vi "LS330_AddArray.vi"(9 "Array Cluster IN":T2, 10 "Queue IN":T4) -> (1 "Array Cluster OUT":T2, 2 "XY Plot Data":T1(array[cluster]))   [LabVIEW 2021]
uses:
  LS330_Status_Bundle.ctl
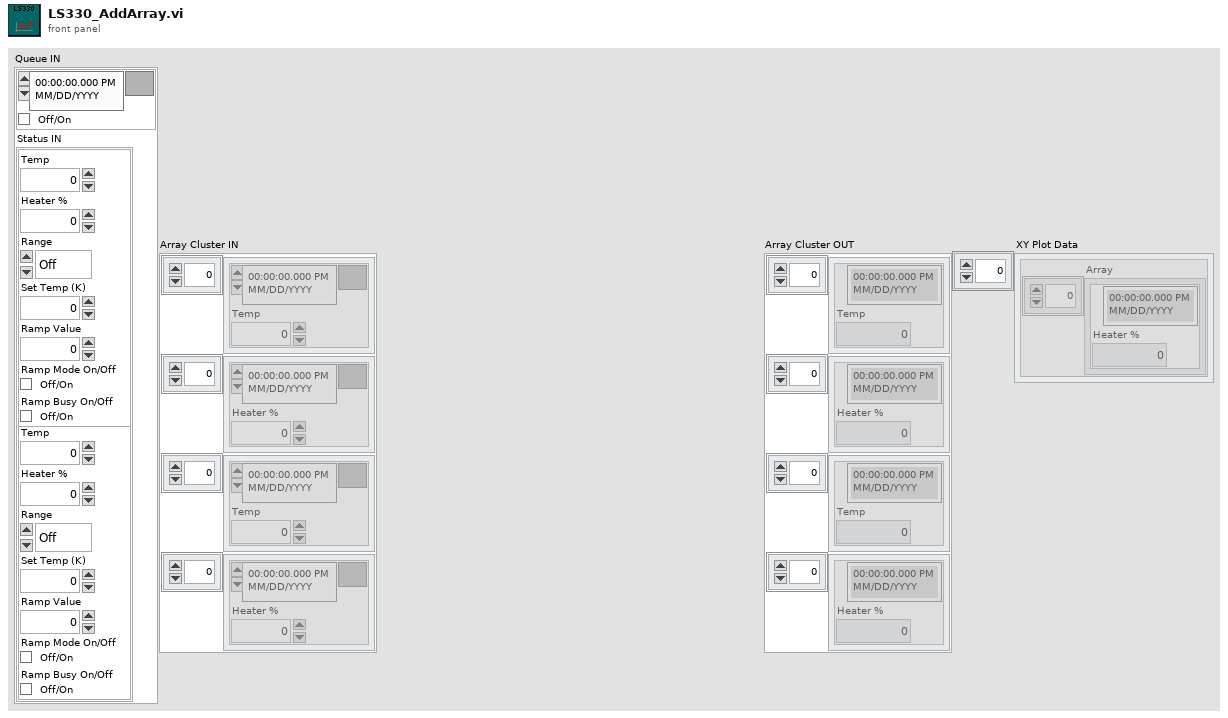
[diagram p1: front panel]
types:
  T1 = cluster{"Array":cluster{timestamp, "Heater %":dbl}[]}[]
  T2 = cluster{"Array":cluster{timestamp, "Temp":dbl}[], "Array":cluster{timestamp, "Heater %":dbl}[], "Array":cluster{timestamp, "Temp":dbl}[], "Array":cluster{timestamp, "Heater %":dbl}[]}
  T3 = typedef "LS330_Status_Bundle.ctl" = cluster{"Temp":dbl, "Heater %":dbl, "Range":enum16{"Off", "Low", "Medium", "High"}, "Set Temp (K)":dbl, "Ramp Value":dbl, "Ramp Mode On/Off":bool, "Ramp Busy On/Off":bool}
  T4 = cluster{"Cluster":cluster{timestamp, "Checkbox":bool}, "Status IN":cluster{T3, T3}}
  T5 = cluster{"Array":cluster{timestamp, "Temp":dbl}[]}
  T6 = cluster{"Array":cluster{timestamp, "Heater %":dbl}[]}
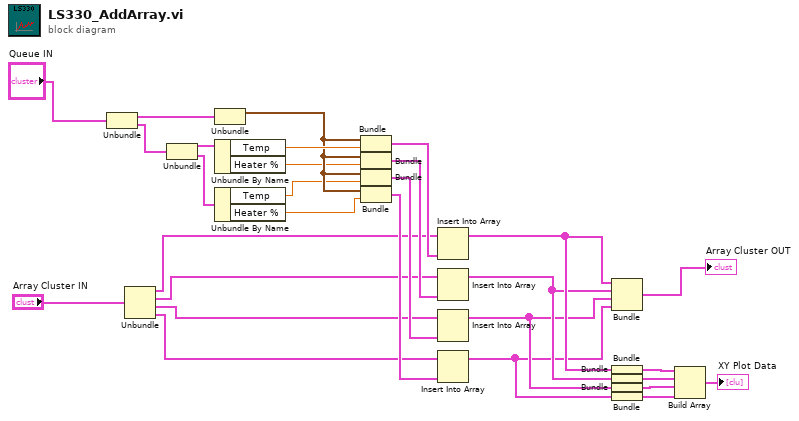
[diagram p0: block diagram]
diagram:
  n1 = Unbundle("Queue IN") -> ("Cluster"=w28:cluster{timestamp, "Checkbox":bool}, "Status IN"=w27:cluster{T3, T3})
  n2 = Unbundle("Array Cluster IN") -> ("Array"=w13:cluster{timestamp, "Temp":dbl}[], "Array"=w12:cluster{timestamp, "Heater %":dbl}[], "Array"=w11:cluster{timestamp, "Temp":dbl}[], "Array"=w10:cluster{timestamp, "Heater %":dbl}[])
  n3 = Unbundle(w27) -> (w26:T3, w25:T3)
  n4 = Unbundle(w28) -> (w23:timestamp)  [unwired: 1 out]
  n5 = Unbundle By Name(w26) -> ("Temp"=w24:dbl, "Heater %"=w22:dbl)
  n6 = Unbundle By Name(w25) -> ("Temp"=w21:dbl, "Heater %"=w20:dbl)
  n7 = Bundle(w23, "Temp"=w24) -> (w19:cluster{timestamp, "Temp":dbl})  [unwired: 1 in]
  n8 = Bundle(w23, "Heater %"=w22) -> (w18:cluster{timestamp, "Heater %":dbl})  [unwired: 1 in]
  n9 = Bundle(w23, "Temp"=w21) -> (w17:cluster{timestamp, "Temp":dbl})  [unwired: 1 in]
  n10 = Bundle(w23, "Heater %"=w20) -> (w16:cluster{timestamp, "Heater %":dbl})  [unwired: 1 in]
  n11 = Insert Into Array(array=w13, new element=w19) -> (w9:cluster{timestamp, "Temp":dbl}[])  [unwired: 1 in]
  n12 = Insert Into Array(array=w12, new element=w18) -> (w8:cluster{timestamp, "Heater %":dbl}[])  [unwired: 1 in]
  n13 = Insert Into Array(array=w11, new element=w17) -> (w7:cluster{timestamp, "Temp":dbl}[])  [unwired: 1 in]
  n14 = Insert Into Array(array=w10, new element=w16) -> (w6:cluster{timestamp, "Heater %":dbl}[])  [unwired: 1 in]
  n15 = Bundle("Array"=w9, "Array"=w8, "Array"=w7, "Array"=w6) -> (→"Array Cluster OUT":T2)  [unwired: 1 in]
  n16 = Bundle("Array"=w9) -> (w5:T5)  [unwired: 1 in]
  n17 = Bundle("Array"=w8) -> (w4:T6)  [unwired: 1 in]
  n18 = Bundle("Array"=w7) -> (w3:T5)  [unwired: 1 in]
  n19 = Bundle("Array"=w6) -> (w2:T6)  [unwired: 1 in]
  n20 = Build Array(w5, w4, w3, w2) -> (→"XY Plot Data":T1)
